vi "6700C Wrapper.vi"(5 "DUT":string, 6 "Measurement Type":i32(ring)=1 items=["Current", "Voltage", "Power"], 7 "States":T2, 8 "error in":errorcluster, 9 "Enable Output":bool, 10 "Setting":T1={"Max Volt"=10.0, "Voltage Set"=0.01, "Current Lim"=0.5}, 11 "Alias":string="PS1") -> (0 "error out":errorcluster, 3 "Measurement":dbl=nan)   [LabVIEW 2021, in "MIO Wrappers.lvlib"]
doc: "This is a wrapper to support Keysight N6700C."
uses:
  MIO Wrappers.lvlib
  <instrlib>/Agilent N6700 Series/Agilent N6700 Series.lvlib
  Load INI/Controls/Instruments_Data.ctl
  09cf5d2b-2ff2-4268-86fd-4cb5ec4a1ae2.vi
  Controls/PS States.ctl
panel:
  # "This wrapper has only been tested with N6773A and\nN6744B PS Modules (loaded in N6700C mainframe\nall other models are disabled unless tested and added to list"
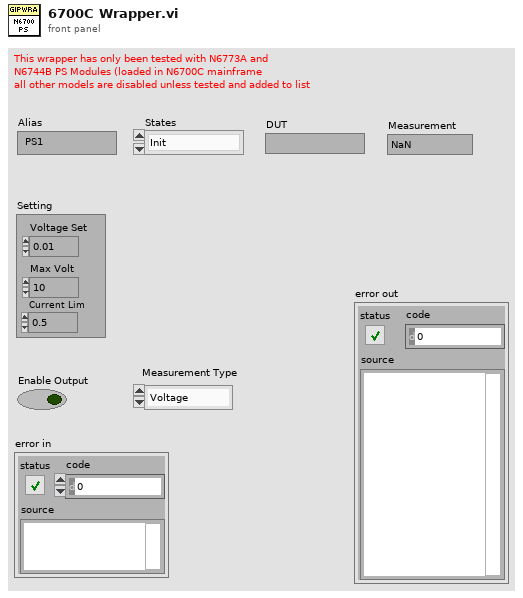
[diagram p1: front panel]
types:
  T1 = cluster{"Max Volt":dbl, "Voltage Set":dbl, "Current Lim":dbl}
  T2 = typedef "MIO Wrappers.lvlib/PS States.ctl" = enum16{"Init", "Config", "Enable Output", "Measure", "Close"}
  T3 = typedef "Instruments_Data.ctl" = cluster{"Alias":string, "Resource ":string}
  T4 = cluster{"Channel Name":string, "VISA resource name":refnum<visa-resource-name>}
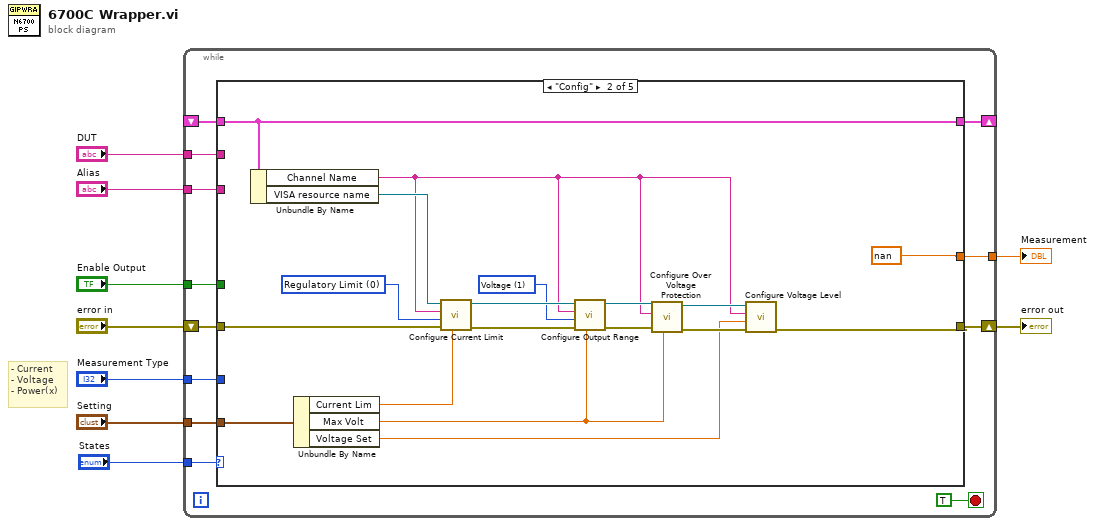
[diagram p0: block diagram]
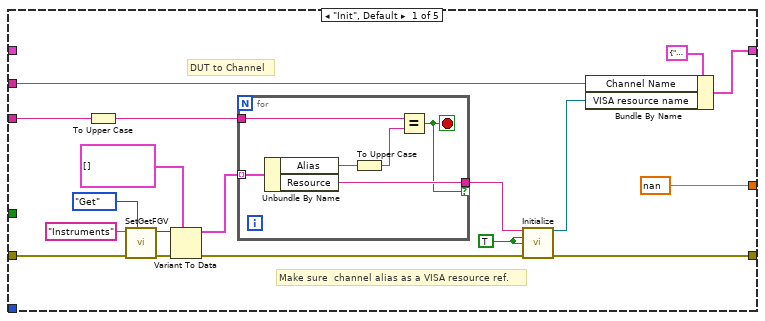
[diagram p2: hidden frame]
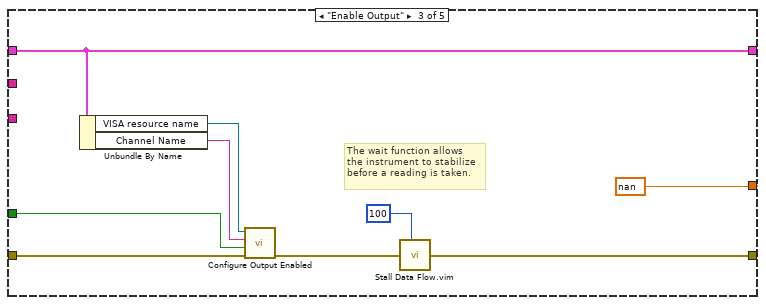
[diagram p3: hidden frame]
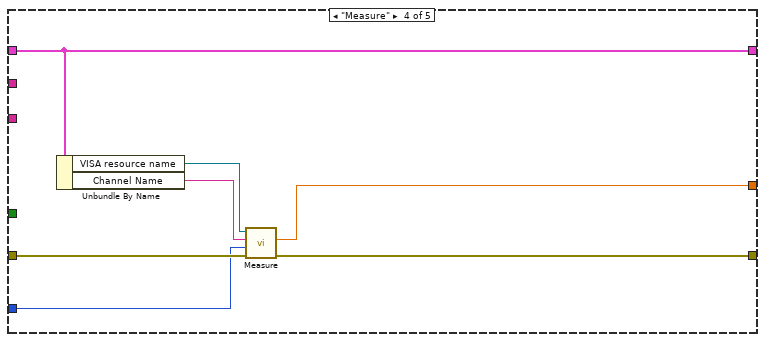
[diagram p4: hidden frame]
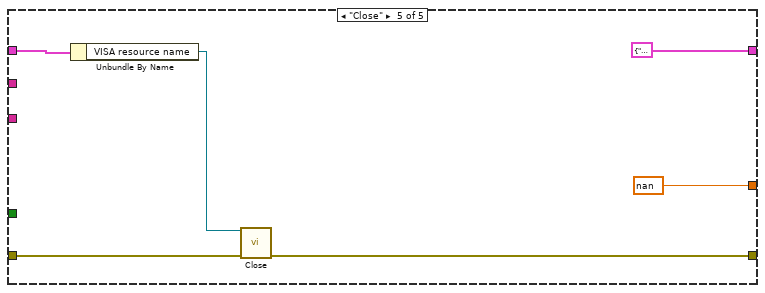
[diagram p5: hidden frame]
diagram:
  # "- Current\n- Voltage\n- Power(x)"
  n1 = while {
    tunnel: "States" -> [w20]
    tunnel: "Enable Output" -> [w18]
    tunnel: "Setting" -> [w17]
    tunnel: "Alias" -> [w16]
    tunnel: [w15] -> w3
    tunnel: "Measurement Type" -> [w14]
    tunnel: "DUT" -> [w13]
    shift-right: [w19] -> w7
    shift-left: "error in" -> [w21]
    shift-right: [w11] -> _
    shift-left: _ -> [w10]
    stop <- TRUE stop-if-true
    n2 = case shown="\"Config\"" w20 {
      tunnel: w21 -> [w37 w52 w72 w76 w82]
      tunnel: [w24 w60 w65 w78 w80] -> w19
      tunnel: [w38 w63 w71 w77 T4 {"Channel Name"="", "VISA resource name"=""}] -> w11
      tunnel: w10 -> [_ w63 w71 w77 w85]
      tunnel: [nan nan nan w79 nan] -> w15
      tunnel: w18 -> [_ _ w69 _ _]
      tunnel: w17 -> [_ w62 _ _ _]
      tunnel: w16 -> [w31 _ _ _ _]
      tunnel: w14 -> [_ _ _ w73 _]
      tunnel: w13 -> [w22 _ _ _ _]
      frame "Init", Default {
        w28 = TRUE ("Reset? (T: Yes)")
        # "DUT to Channel"
        # "Make sure  channel alias as a VISA resource ref."
        # "Initialize and create VISA resource ref from INI mapper"
        n3 = To Upper Case(1:w31) -> (0:w30:string)
        n4 = call "SetGetFGV.vi"("Method (Get)"=enum16{"Get", "Set"}."Get", "error in"=w37, "FGVname"="Instruments" ("Name")) -> ("error out"=w35:errorcluster, "Data out"=w34:variant)  [unwired: 7 in]
        n5 = Variant To Data(error in=w35, type=T3[] [], Variant=w34) -> (data=w32:T3[], error out=w25:errorcluster)
        n6 = for {
          tunnel: w32 -> [w45] mode=indexing
          tunnel: w30 -> [w44]
          tunnel: [w41] -> w29 if=w40
          stop <- w40 stop-if-true
          n7 = Unbundle By Name(w45) -> ("Alias"=w42:string, "Resource"=w41:string)
          n8 = To Upper Case(1:w42) -> (0:w43:string)
          n9 = Equal?(x=w44, y=w43) -> (x = y?=w40:bool)
        }
        n10 = call <instrlib>:"Initialize.vi"("VISA resource name"=w29, "ID Query? (T: Yes)"=w28, "Reset? (T: Yes)"=w28, "error in (no error)"=w25) -> ("VISA resource name out"=w23:refnum<visa-resource-name>, "error out"=w24:errorcluster)  [unwired: 10 in]
        n11 = Bundle By Name(cluster=T4 {"Channel Name"="", "VISA resource name"=""}, "Channel Name"=w22, "VISA resource name"=w23) -> (w38:T4)
      }
      frame "Config" {
        w46 = 1 items=["Voltage"=1, "Current"=0] ("Range Type (1: Voltage)")
        w57 = 0 items=["Regulatory Limit", "Trip Limit"] ("Behavior (0: Regulatory Limit)")
        n12 = Unbundle By Name(w63) -> ("Channel Name"=w47:string, "VISA resource name"=w53:refnum<visa-resource-name>)
        n13 = Unbundle By Name(w62) -> ("Current Lim"=w59:dbl, "Max Volt"=w58:dbl, "Voltage Set"=w54:dbl)
        n14 = call <instrlib>:"Configure Current Limit.vi"("Limit (0.0 amps)"=w59, "error in (no error)"=w52, "Behavior (0: Regulatory Limit)"=w57, "Channel Name (1)"=w47, "VISA resource name"=w53) -> ("error out"=w50:errorcluster, "VISA resource name out"=w51:refnum<visa-resource-name>)  [unwired: 5 in]
        n15 = call <instrlib>:"Configure Output Range.vi"("Range (0.0)"=w58, "error in (no error)"=w50, "Range Type (1: Voltage)"=w46, "Channel Name (1)"=w47, "VISA resource name"=w51) -> ("error out"=w49:errorcluster, "VISA resource name out"=w48:refnum<visa-resource-name>)  [unwired: 5 in]
        n16 = call <instrlib>:"Configure Over Voltage Protection.vi"("Limit (0.0 volts)"=w58, "error in (no error)"=w49, "Channel Name (1)"=w47, "VISA resource name"=w48) -> ("error out"=w55:errorcluster, "VISA resource name out"=w56:refnum<visa-resource-name>)  [unwired: 6 in]
        n17 = call <instrlib>:"Configure Voltage Level.vi"("error in (no error)"=w55, "Level  (0.0 volts)"=w54, "Channel Name (1)"=w47, "VISA resource name"=w56) -> ("error out"=w60:errorcluster)  [unwired: 6 in, 1 out]
      }
      frame "Enable Output" {
        # "The wait function allows \nthe instrument to stabilize\nbefore a reading is taken."
        n18 = Unbundle By Name(w71) -> ("VISA resource name"=w68:refnum<visa-resource-name>, "Channel Name"=w70:string)
        n19 = call <instrlib>:"Configure Output Enabled.vi"("error in (no error)"=w72, "Enable Output (False)"=w69, "Channel Name (1)"=w70, "VISA resource name"=w68) -> ("error out"=w67:errorcluster)  [unwired: 6 in, 1 out]
        n20 = call "Stall Data Flow.vim"("value in"=w67, "milliseconds to wait"=u32 100) -> ("value out"=w65:errorcluster)  [unwired: 1 out]
      }
      frame "Measure" {
        n21 = Unbundle By Name(w77) -> ("VISA resource name"=w75:refnum<visa-resource-name>, "Channel Name"=w74:string)
        n22 = call <instrlib>:"Measure.vi"("error in (no error)"=w76, "Measurement Type (1: Voltage)"=w73, "Channel Name (1)"=w74, "VISA resource name"=w75) -> ("error out"=w78:errorcluster, "Measurement"=w79:dbl)  [unwired: 5 in, 1 out]
      }
      frame "Close" {
        n23 = Unbundle By Name(w85) -> ("VISA resource name"=w81:refnum<visa-resource-name>)
        n24 = call <instrlib>:"Close.vi"("VISA resource name"=w81, "error in (no error)"=w82) -> ("error out"=w80:errorcluster)  [unwired: 13 in]
      }
    }
  }
  "error out" <- w7
  "Measurement" <- w3
